vi "SubVI_Define_local.vi"(7 "QRCode":bool, 8 "Cluster C":T2, 9 "Cluster B":T2, 10 "Cluster A":T2, 11 "Linha da tabela":string[](array[string])) -> (1 "Destino":string, 2 "Local destino":T1(ring))   [LabVIEW 2017]
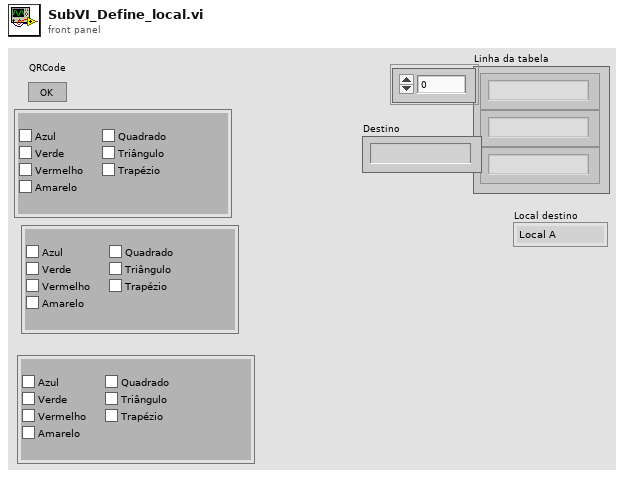
[diagram p1: front panel]
types:
  T1 = enum16{"Local A", "Local B", "Local C", "Discard"}
  T2 = cluster{"Azul":bool, "Verde":bool, "Vermelho":bool, "Amarelo":bool, "Quadrado":bool, "Triângulo":bool, "Trapézio":bool}
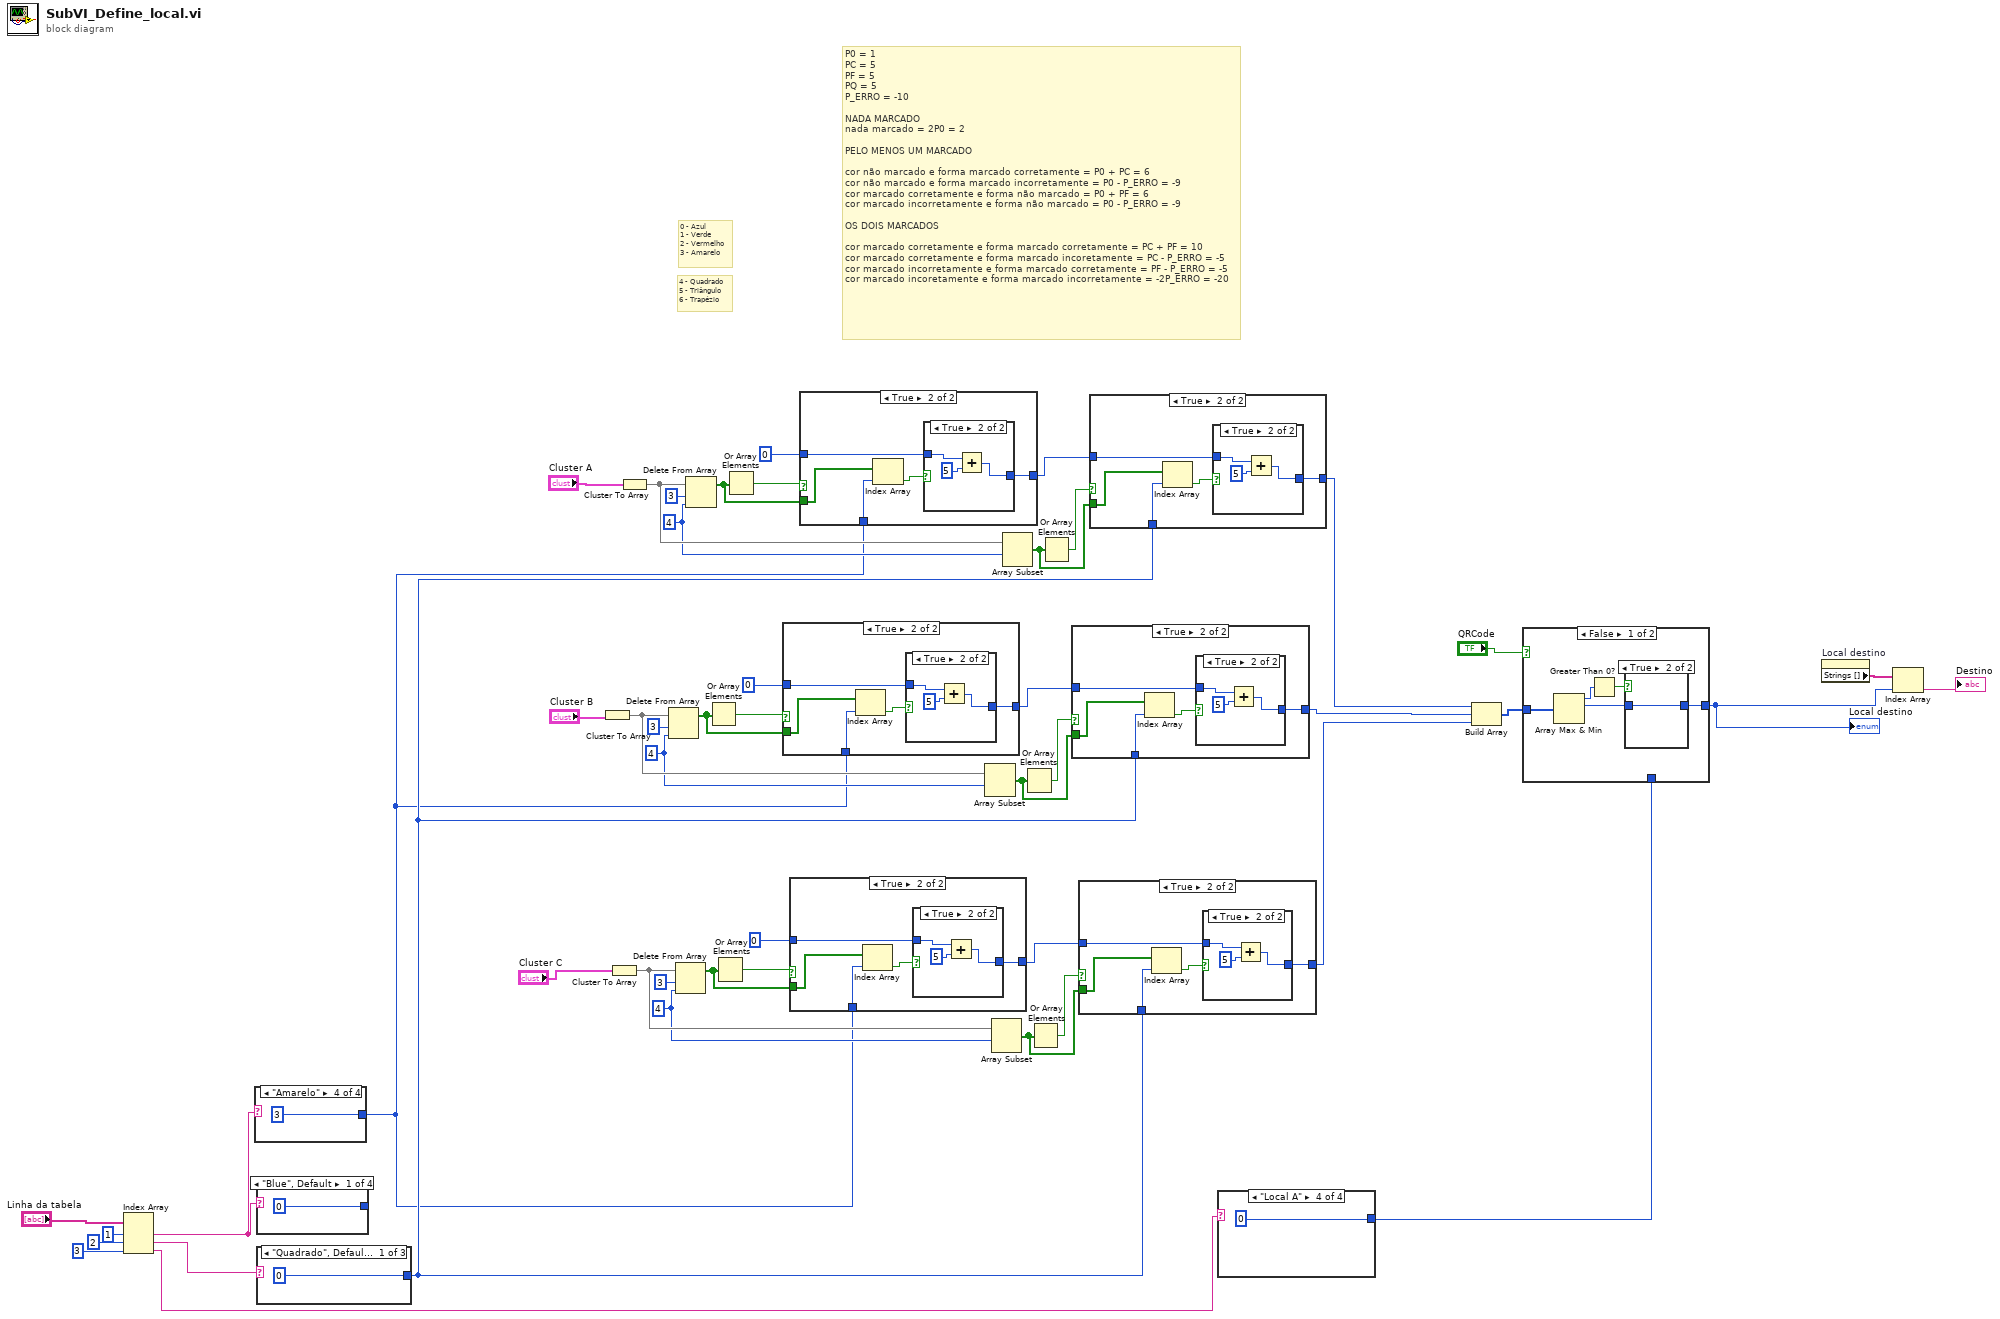
[diagram p0: block diagram]
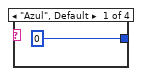
[diagram p2: hidden frame]
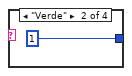
[diagram p3: hidden frame]
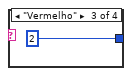
[diagram p4: hidden frame]
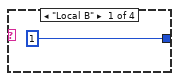
[diagram p5: hidden frame]
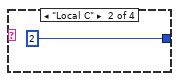
[diagram p6: hidden frame]
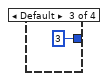
[diagram p7: hidden frame]
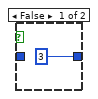
[diagram p8: hidden frame]
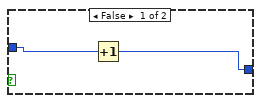
[diagram p10: hidden frame]
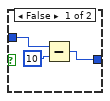
[diagram p11: hidden frame]
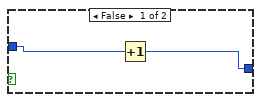
[diagram p12: hidden frame]
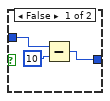
[diagram p13: hidden frame]
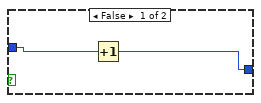
[diagram p14: hidden frame]
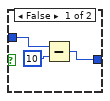
[diagram p15: hidden frame]
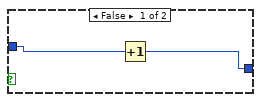
[diagram p16: hidden frame]
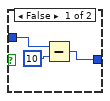
[diagram p17: hidden frame]
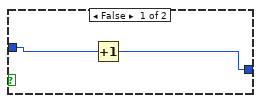
[diagram p18: hidden frame]
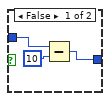
[diagram p19: hidden frame]
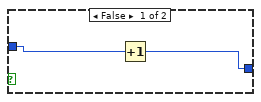
[diagram p20: hidden frame]
diagram:
  w21 = 4 ("index")
  w31 = 4 ("index")
  w42 = 4 ("index")
  # "P0 = 1\nPC = 5\nPF = 5\nPQ = 5\nP_ERRO = -10\n\nNADA MARCADO\nnada marcado = 2P0 = 2\n\nPELO MENOS UM MARCADO\n\ncor não marcado e forma marcado corretamente = P0 + PC = 6\ncor não marcado e forma marcado incorretamente = P0 - P_ERRO = -9\ncor marcado corretamente e forma não marcado = P0 + PF = 6\ncor marcado incorretamente e forma não marcado = P0 - P_ERRO = -9\n\nOS DOIS MARCADOS\n\ncor marcado corretamente e forma marcado corretamente = PC + PF = 10\ncor marcado corretamente e forma marcado incoretamente = PC - P_ERRO = -5\ncor marcado incorretamente e forma marcado corretamente = PF - P_ERRO = -5\ncor marcado incoretamente e forma marcado incorretamente = -2P_ERRO = -20"
  # "4 - Quadrado\n5 - Triângulo\n6 - Trapézio"
  # "0 - Azul\n1 - Verde\n2 - Vermelho\n3 - Amarelo"
  n1 = Index Array(array="Linha da tabela", index #1=1 ("index"), index #2=2 ("index"), index #3=3 ("index")) -> (element #1=w2:string, element #2=w41:string, element #3=w5:string)
  n2 = case shown="\"Amarelo\"" w2 {
    tunnel: [0 1 2 3] -> w1
    frame "Azul", Default {
    }
    frame "Verde" {
    }
    frame "Vermelho" {
    }
    frame "Amarelo" {
    }
  }
  n3 = case shown="\"Blue\", Default" w2 {
    tunnel: [0 1 2 3] -> _
    frame "Blue", Default {
    }
    frame "Green" {
    }
    frame "Red" {
    }
    frame "Yellow" {
    }
  }
  n4 = case shown="\"Quadrado\", Default" w41 {
    tunnel: [0 1 2] -> w13
    frame "Quadrado", Default {
    }
    frame "Triângulo" {
    }
    frame "Trapézio" {
    }
  }
  n5 = Cluster To Array(cluster="Cluster B") -> (array=w32:bool[])
  n6 = Cluster To Array(cluster="Cluster C") -> (array=w22:bool[])
  n7 = Cluster To Array(cluster="Cluster A") -> (array=w43:bool[])
  n8 = Delete From Array(array=w32, length=3, index=w31) -> (array with subset deleted=w28:bool[])  [unwired: 1 out]
  n9 = Delete From Array(array=w22, length=3, index=w21) -> (array with subset deleted=w18:bool[])  [unwired: 1 out]
  n10 = Delete From Array(array=w43, length=3, index=w42) -> (array with subset deleted=w38:bool[])  [unwired: 1 out]
  n11 = Or Array Elements(Boolean array=w28) -> (logical OR=w30:bool)
  n12 = Or Array Elements(Boolean array=w18) -> (logical OR=w20:bool)
  n13 = Or Array Elements(Boolean array=w38) -> (logical OR=w40:bool)
  n14 = case shown="True" w30 {
    tunnel: 0 -> [w61 w63]
    tunnel: [w60 w62] -> w27
    tunnel: w1 -> [_ w65]
    tunnel: w28 -> [_ w66]
    frame False {
      n15 = Increment(x=w61) -> (x+1=w60:i32)
    }
    frame True {
      n16 = Index Array(array=w66, index=w65) -> (element=w64:bool)
      n17 = case shown="True" w64 {
        tunnel: w63 -> [w68 w72]
        tunnel: [w69 w70] -> w62
        frame False {
          n18 = Subtract(x=w68, y=10) -> (x-y=w69:i32)
        }
        frame True {
          n19 = Add(x=w72, y=5) -> (x+y=w70:i32)
        }
      }
    }
  }
  n20 = case shown="True" w20 {
    tunnel: 0 -> [w74 w76]
    tunnel: [w73 w75] -> w17
    tunnel: w1 -> [_ w78]
    tunnel: w18 -> [_ w79]
    frame False {
      n21 = Increment(x=w74) -> (x+1=w73:i32)
    }
    frame True {
      n22 = Index Array(array=w79, index=w78) -> (element=w77:bool)
      n23 = case shown="True" w77 {
        tunnel: w76 -> [w81 w85]
        tunnel: [w82 w83] -> w75
        frame False {
          n24 = Subtract(x=w81, y=10) -> (x-y=w82:i32)
        }
        frame True {
          n25 = Add(x=w85, y=5) -> (x+y=w83:i32)
        }
      }
    }
  }
  n26 = case shown="True" w40 {
    tunnel: 0 -> [w87 w89]
    tunnel: [w86 w88] -> w37
    tunnel: w1 -> [_ w91]
    tunnel: w38 -> [_ w92]
    frame False {
      n27 = Increment(x=w87) -> (x+1=w86:i32)
    }
    frame True {
      n28 = Index Array(array=w92, index=w91) -> (element=w90:bool)
      n29 = case shown="True" w90 {
        tunnel: w89 -> [w94 w98]
        tunnel: [w95 w96] -> w88
        frame False {
          n30 = Subtract(x=w94, y=10) -> (x-y=w95:i32)
        }
        frame True {
          n31 = Add(x=w98, y=5) -> (x+y=w96:i32)
        }
      }
    }
  }
  n32 = Array Subset(array=w32, index=w31) -> (w26:bool[])  [unwired: 1 in]
  n33 = Array Subset(array=w22, index=w21) -> (w16:bool[])  [unwired: 1 in]
  n34 = Array Subset(array=w43, index=w42) -> (w36:bool[])  [unwired: 1 in]
  n35 = Or Array Elements(Boolean array=w26) -> (logical OR=w25:bool)
  n36 = Or Array Elements(Boolean array=w16) -> (logical OR=w15:bool)
  n37 = Or Array Elements(Boolean array=w36) -> (logical OR=w35:bool)
  n38 = case shown="True" w25 {
    tunnel: w27 -> [w100 w102]
    tunnel: [w99 w101] -> w23
    tunnel: w13 -> [_ w104]
    tunnel: w26 -> [_ w105]
    frame False {
      n39 = Increment(x=w100) -> (x+1=w99:i32)
    }
    frame True {
      n40 = Index Array(array=w105, index=w104) -> (element=w103:bool)
      n41 = case shown="True" w103 {
        tunnel: w102 -> [w107 w111]
        tunnel: [w108 w109] -> w101
        frame False {
          n42 = Subtract(x=w107, y=10) -> (x-y=w108:i32)
        }
        frame True {
          n43 = Add(x=w111, y=5) -> (x+y=w109:i32)
        }
      }
    }
  }
  n44 = case shown="True" w15 {
    tunnel: w17 -> [w113 w115]
    tunnel: [w112 w114] -> w12
    tunnel: w13 -> [_ w117]
    tunnel: w16 -> [_ w118]
    frame False {
      n45 = Increment(x=w113) -> (x+1=w112:i32)
    }
    frame True {
      n46 = Index Array(array=w118, index=w117) -> (element=w116:bool)
      n47 = case shown="True" w116 {
        tunnel: w115 -> [w120 w124]
        tunnel: [w121 w122] -> w114
        frame False {
          n48 = Subtract(x=w120, y=10) -> (x-y=w121:i32)
        }
        frame True {
          n49 = Add(x=w124, y=5) -> (x+y=w122:i32)
        }
      }
    }
  }
  n50 = case shown="True" w35 {
    tunnel: w37 -> [w126 w128]
    tunnel: [w125 w127] -> w33
    tunnel: w13 -> [_ w130]
    tunnel: w36 -> [_ w131]
    frame False {
      n51 = Increment(x=w126) -> (x+1=w125:i32)
    }
    frame True {
      n52 = Index Array(array=w131, index=w130) -> (element=w129:bool)
      n53 = case shown="True" w129 {
        tunnel: w128 -> [w133 w137]
        tunnel: [w134 w135] -> w127
        frame False {
          n54 = Subtract(x=w133, y=10) -> (x-y=w134:i32)
        }
        frame True {
          n55 = Add(x=w137, y=5) -> (x+y=w135:i32)
        }
      }
    }
  }
  n56 = case shown="\"Local A\"" w5 {
    tunnel: [1 2 3 0] -> w3
    frame "Local B" {
    }
    frame "Local C" {
    }
    frame Default {
    }
    frame "Local A" {
    }
  }
  n57 = Build Array(w33, w23, w12) -> (w34:i32[])
  n58 = case shown="False" "QRCode" {
    tunnel: w34 -> [w146 _]
    tunnel: [w142 w149] -> w10
    tunnel: w3 -> [_ w149]
    frame False {
      n59 = Array Max & Min(array=w146) -> (max value=w144:i32, max index (indices)=w143:i32)  [unwired: 2 out]
      n60 = Greater Than 0?(x=w144) -> (x > 0?=w145:bool)
      n61 = case shown="True" w145 {
        tunnel: w143 -> [_ w148]
        tunnel: [3 w148] -> w142
        frame False {
        }
        frame True {
        }
      }
    }
    frame True {
    }
  }
  "Local destino" <- w10
  n62 = property on="Local destino" class="Enum (strict)"() -> ("Strings []"=w11:string[])  [unwired: 2 in, 2 out]
  n63 = Index Array(array=w11, index=w10) -> (element=→"Destino":string)
